vi "Configure Signal Route.vi"(8 "error in (no error)":errorcluster, 9 "Signal (0: Marker 1)":i32(ring) items=["Marker 1", "Marker 2", "Marker 3", "Marker 4", "None", "Sweep Out", "Source Settled", "Pulse Video", "Pulse Sync", "Sweep Out for 8757D", "Sweep Run", "Swept Function Done", "LXI", "Pulse", "AUX29", "TRIG2", "TRIG1"], 10 "Connector (0: PAT TRIG)":i32(ring) items=["PAT TRIG", "BB TRIG 1", "BB TRIG 2", "SWEEP OUT", "TRIG 1", "TRIG 2"], 11 "VISA resource name":refnum<visa-resource-name>) -> (0 "error out":errorcluster, 3 "VISA resource name out":refnum<visa-resource-name>)   [LabVIEW 2018, in "Agilent PSG MXG Series.lvlib"]
doc: "Specifies the signal-connector routing policy.\n\n<B>Notes:</B>\n(1) This VI is valid only in N5171B, N5181B, N5172B, N5182B, N5173B, N5183B.\n\n(2) For N5172B, this VI is valid only when the instrument installs <B>Option 653</B> or <B>Option 655</B>.\n\n(3) For N5182B, this VI is valid only when the instrument installs <B>Option 656</B> or <B>Option 657</B>."
uses:
  Agilent PSG MXG Series.lvlib
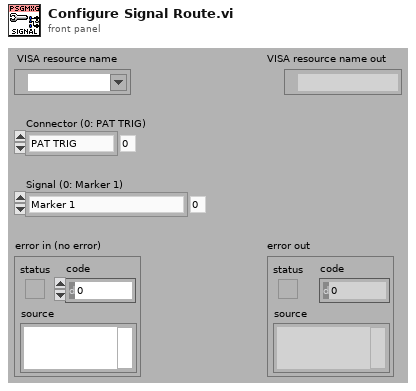
[diagram p1: front panel]
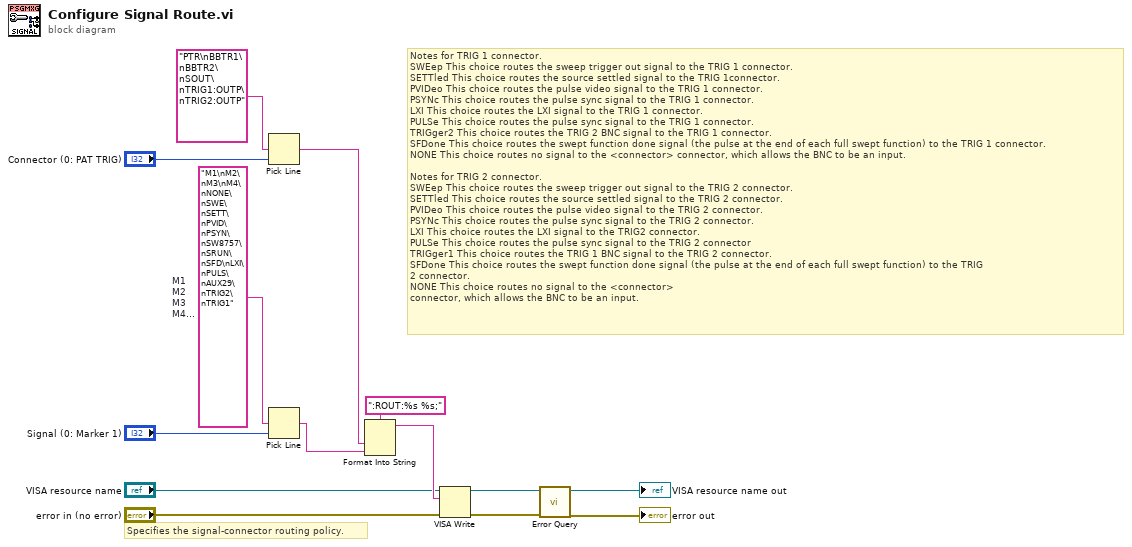
[diagram p0: block diagram]
diagram:
  w12 = "M1\nM2\nM3\nM4\nNONE\nSWE\nSETT\nPVID\nPSYN\nSW8757\nSRUN\nSFD\nLXI\nPULS\nAUX29\nTRIG2\nTRIG1"  # M1 M2 M3 M4 NONE SWE SETT PVID PSYN SW8757 SRUN SFD LXI PULS AUX29 TRIG2 TRIG1
  # "Notes for TRIG 1 connector.\nSWEep This choice routes the sweep trigger out signal to the TRIG 1 connector.\nSETTled This choice routes the source settled signal to the TRIG 1connector.\nPVIDeo This choice routes the pulse video signal to the TRIG 1 connector.\nPSYNc This choice routes the pulse sync signal to the TRIG 1 connector.\nLXI This choice routes the LXI signal to the TRIG 1 connector.\nPULSe This choice routes the pulse sync signal to the TRIG 1 connector.\nTRIGger2 This choice routes the TRIG 2 BNC signal to the TRIG 1 connector.\nSFDone This choice routes the swept function done signal (the pulse at the end of each full swept function) to the TRIG 1 connector.\nNONE This choice routes no signal to the <connector> connector, which allows the BNC to be an input.\n\nNotes for TRIG 2 connector.\nSWEep This choice routes the sweep trigger out signal to the TRIG 2 connector.\nSETTled This choice routes the source settled signal to the TRIG 2 connector.\nPVIDeo This choice routes the pulse video signal to the TRIG 2 connector.\nPSYNc This choice routes the pulse sync signal to the TRIG 2 connector.\nLXI This choice routes the LXI signal to the TRIG2 connector.\nPULSe This choice routes the pulse sync signal to the TRIG 2 connector\nTRIGger1 This choice routes the TRIG 1 BNC signal to the TRIG 2 connector.\nSFDone This choice routes the swept function done signal (the pulse at the end of each full swept function) to the TRIG\n2 connector.\nNONE This choice routes no signal to the <connector>\nconnector, which allows the BNC to be an input."
  # "Specifies the signal-connector routing policy."
  n1 = Pick Line(multi-line string="PTR\nBBTR1\nBBTR2\nSOUT\nTRIG1:OUTP\nTRIG2:OUTP", line index="Connector (0: PAT TRIG)") -> (output string=w9:string)  [unwired: 1 out]
  n2 = Pick Line(multi-line string=w12, line index="Signal (0: Marker 1)") -> (output string=w8:string)  [unwired: 1 out]
  n3 = Format Into String(format string=":ROUT:%s %s;", w9, w8) -> (resulting string=w7:string)  [unwired: 2 in, 1 out]
  n4 = VISA Write(VISA resource name="VISA resource name", write buffer=w7, error in (no error)="error in (no error)") -> (VISA resource name out=w4:refnum<visa-resource-name>, error out=w3:errorcluster)  [unwired: 1 out]
  n5 = call "Error Query.vi"("error in (no error)"=w3, "VISA resource name"=w4) -> ("error out"=→"error out":errorcluster, "VISA resource name out"=→"VISA resource name out":refnum<visa-resource-name>)  [unwired: 8 out]
